vi "Mouvement encodeur.vi"(6 "Vitesse initiale":dbl, 7 "Temps acceleration":dbl, 8 "Reverse":bool, 9 "Left":bool, 10 "Right":bool, 11 "Distance":dbl) -> ()   [LabVIEW 2016]
uses:
  <vilib>/Rock Robotics/WPI/Utilities/WPI_GetSetVariantRefNum.vi
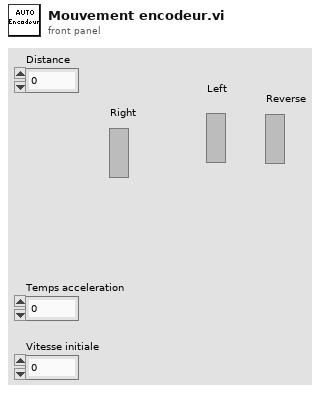
[diagram p1: front panel]
types:
  T1 = typedef "WPI_EncoderDevRef.ctl" = cluster{"DevStatus":errorcluster, "EncoderIndex":T2, "CounterIndex":T3, "DistancePerCount":dbl, "Decoding Type":T4}
  T2 = typedef "FPGA_EncoderIdx.ctl" = enum8{"Enc 0", "Enc 1", "Enc 2", "Enc 3", "Enc 4", "Enc 5", "Enc 6", "Enc 7", "Invalid"}
  T3 = typedef "FPGA_CounterCtrSystemIndex.ctl" = enum8{"Ctr 0", "Ctr 1", "Ctr 2", "Ctr 3", "Ctr 4", "Ctr 5", "Ctr 6", "Ctr 7", "Invalid"}
  T4 = typedef "WPI_EncoderType.ctl" = enum16{"1x", "2x", "4x"}
  T5 = typedef "WPI_RobotDriveDevRef.ctl" = cluster{"DevStatus":errorcluster, "Motors[]":T6[], "Square Inputs":bool, "Max Output":dbl}
  T6 = typedef "WPI_MotorControlDeviceRef.ctl" = cluster{"DeviceStatus":errorcluster, "Type":T7, "PWM":cluster{"PWM Channel":T8, "DeadBand":T9}, "CAN":cluster{"Device Number":u8, "SetOutput VI Ref":variant, "GetOutput VI Ref":variant, "Enable VI Ref":variant, "Disable VI Ref":variant, "Data":variant}, "Invert":bool}
  T7 = typedef "WPI_MotorControlType.ctl" = enum16{"PWM", "CAN"}
  T8 = typedef "FPGA_DIOPWMChannel.ctl" = enum8{"PWM 0", "PWM 1", "PWM 2", "PWM 3", "PWM 4", "PWM 5", "PWM 6", "PWM 7", "PWM 8", "PWM 9", "PWM MXP 0", "PWM MXP 1", "PWM MXP 2", "PWM MXP 3", "PWM MXP 4", "PWM MXP 5", "PWM MXP 6", "PWM MXP 7", "PWM MXP 8", "PWM MXP 9", "Invalid"}
  T9 = typedef "WPI_PWMDeadband.ctl" = cluster{"Name":string, "maxPositivePwm":i32, "minPositivePwm":i32, "centerPwm":i32, "maxNegativePwm":i32, "minNegativePwm":i32, "angularRange":u16}
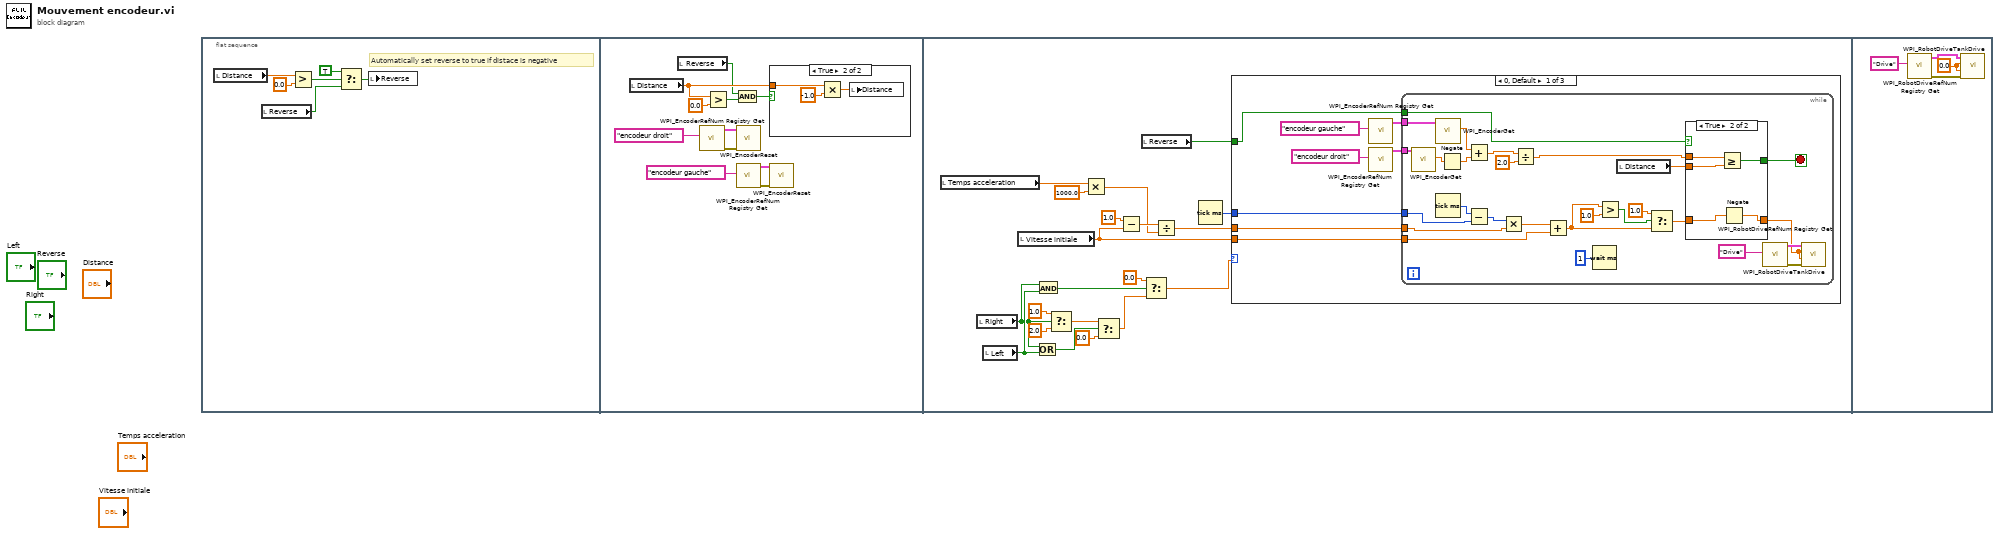
[diagram p0: block diagram]
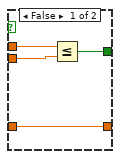
[diagram p3: hidden frame]
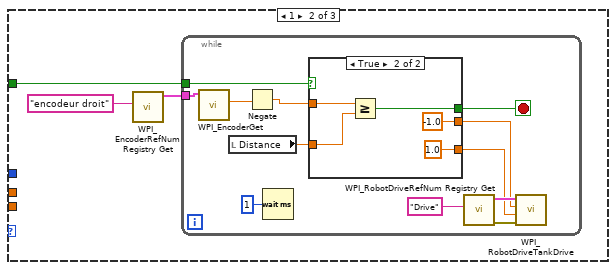
[diagram p4: hidden frame]
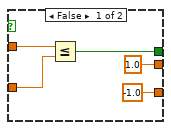
[diagram p5: hidden frame]
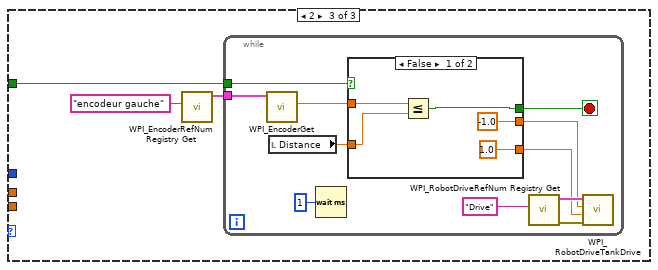
[diagram p6: hidden frame]
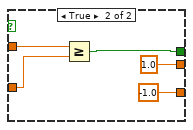
[diagram p7: hidden frame]
diagram:
  n1 = flat-sequence {
    frame #0 {
      # "Automatically set reverse to true if distace is negative"
      n2 = local read "Distance"() -> (w5:dbl)
      n3 = local read "Reverse"() -> (w3:bool)
      n4 = Greater?(x=w5, y=0.0) -> (0:w4:bool)
      n5 = Select(t=TRUE, s=w4, f=w3) -> (s? t:f=w1:bool)
      n6 = local write "Reverse"(w1) -> ()
    }
    frame #1 {
      n7 = local read "Distance"() -> (w11:dbl)
      n8 = local read "Reverse"() -> (w7:bool)
      n9 = call <vilib>:"WPI_EncoderRefNum Registry Get.vi"("refnum name"="encodeur droit") -> ("error out"=w12:errorcluster, "EncoderDevRef"=w13:T1)  [unwired: 9 in]
      n10 = Greater?(x=w11, y=0.0) -> (0:w9:bool)
      n11 = And(x=w7, y=w9) -> (x .and. y?=w10:bool)
      n12 = call <vilib>:"WPI_EncoderReset.vi"("error in (no error)"=w12, "EncoderDevRef"=w13) -> ()  [unwired: 8 in, 2 out]
      n13 = call <vilib>:"WPI_EncoderRefNum Registry Get.vi"("refnum name"="encodeur gauche") -> ("error out"=w14:errorcluster, "EncoderDevRef"=w15:T1)  [unwired: 9 in]
      n14 = case shown="True" w10 {
        tunnel: w11 -> [_ w20]
        frame False {
        }
        frame True {
          n15 = Multiply(x=w20, y=-1.0) -> (x*y=w18:dbl)
          n16 = local write "Distance"(w18) -> ()
        }
      }
      n17 = call <vilib>:"WPI_EncoderReset.vi"("error in (no error)"=w14, "EncoderDevRef"=w15) -> ()  [unwired: 8 in, 2 out]
    }
    frame #2 {
      n18 = local read "Temps acceleration"() -> (w28:dbl)
      n19 = local read "Right"() -> (w32:bool)
      n20 = local read "Left"() -> (w33:bool)
      n21 = local read "Vitesse initiale"() -> (w21:dbl)
      n22 = Or(x=w32, y=w33) -> (x .or. y?=w34:bool)
      n23 = And(x=w32, y=w33) -> (x .and. y?=w31:bool)
      n24 = Select(t=1.0, s=w32, f=2.0) -> (s? t:f=w38:dbl)
      n25 = Multiply(x=w28, y=1000.0) -> (x*y=w24:dbl)
      n26 = Select(t=w38, s=w34, f=0.0) -> (s? t:f=w35:dbl)
      n27 = Subtract(x=1.0, y=w21) -> (x-y=w25:dbl)
      n28 = local read "Reverse"() -> (w29:bool)
      n29 = Select(t=0.0, s=w31, f=w35) -> (s? t:f=w36:dbl)
      n30 = Divide(x=w25, y=w24) -> (x/y=w22:dbl)
      n31 = Tick Count (ms)() -> (millisecond timer value=w23:u32)
      n32 = case shown="0, Default" w36 {
        tunnel: w29 -> [w44 w85 w110]
        tunnel: w23 -> [w43 _ _]
        tunnel: w22 -> [w42 _ _]
        tunnel: w21 -> [w41 _ _]
        frame 0, Default {
          n33 = call <vilib>:"WPI_EncoderRefNum Registry Get.vi"("refnum name"="encodeur gauche") -> ("EncoderDevRef"=w48:T1)  [unwired: 9 in, 1 out]
          n34 = call <vilib>:"WPI_EncoderRefNum Registry Get.vi"("refnum name"="encodeur droit") -> ("EncoderDevRef"=w47:T1)  [unwired: 9 in, 1 out]
          n35 = while {
            tunnel: w47 -> [w75]
            tunnel: w48 -> [w74]
            tunnel: w44 -> [w67]
            tunnel: w43 -> [w65]
            tunnel: w42 -> [w62]
            tunnel: w41 -> [w60]
            stop <- w69 stop-if-true
            n36 = call <vilib>:"WPI_EncoderGet.vi"("EncoderDevRef"=w75) -> ("Distance"=w54:dbl)  [unwired: 5 in, 5 out]
            n37 = call <vilib>:"WPI_EncoderGet.vi"("EncoderDevRef"=w74) -> ("Distance"=w73:dbl)  [unwired: 5 in, 5 out]
            n38 = Tick Count (ms)() -> (millisecond timer value=w64:u32)
            n39 = Negate(x=w54) -> (-x=w53:dbl)
            n40 = Add(x=w73, y=w53) -> (x+y=w72:dbl)
            n41 = Subtract(x=w64, y=w65) -> (x-y=w63:u32)
            n42 = Multiply(x=w63, y=w62) -> (x*y=w61:dbl)
            n43 = Divide(x=w72, y=2.0) -> (x/y=w70:dbl)
            n44 = Add(x=w61, y=w60) -> (x+y=w57:dbl)
            n45 = Wait (ms)(milliseconds to wait=u32 1) -> ()  [unwired: 1 out]
            n46 = Greater?(x=w57, y=1.0) -> (0:w58:bool)
            n47 = local read "Distance"() -> (w68:dbl)
            n48 = Select(t=1.0, s=w58, f=w57) -> (s? t:f=w56:dbl)
            n49 = case shown="True" w67 {
              tunnel: w70 -> [w79 w84]
              tunnel: [w77 w83] -> w69
              tunnel: w68 -> [w78 w82]
              tunnel: [w76 w81] -> w49
              tunnel: w56 -> [w76 w80]
              frame False {
                n50 = Less Or Equal?(x=w79, y=w78) -> (x <= y?=w77:bool)
              }
              frame True {
                n51 = Greater Or Equal?(x=w84, y=w82) -> (x >= y?=w83:bool)
                n52 = Negate(x=w80) -> (-x=w81:dbl)
              }
            }
            n53 = call <vilib>:"WPI_RobotDriveRefNum Registry Get.vi"("refnum name"="Drive") -> ("error out"=w52:errorcluster, "RobotDriveDevRef"=w51:T5)  [unwired: 9 in]
            n54 = call <vilib>:"WPI_RobotDriveTankDrive.vi"("error in (no error)"=w52, "Right axis value"=w49, "Left axis value"=w49, "RobotDriveDevRef"=w51) -> ()  [unwired: 5 in, 3 out]
          }
        }
        frame 1 {
          n55 = call <vilib>:"WPI_EncoderRefNum Registry Get.vi"("refnum name"="encodeur droit") -> ("EncoderDevRef"=w86:T1)  [unwired: 9 in, 1 out]
          n56 = while {
            tunnel: w86 -> [w99]
            tunnel: w85 -> [w93]
            stop <- w98 stop-if-true
            n57 = call <vilib>:"WPI_EncoderGet.vi"("EncoderDevRef"=w99) -> ("Distance"=w89:dbl)  [unwired: 5 in, 5 out]
            n58 = local read "Distance"() -> (w97:dbl)
            n59 = Negate(x=w89) -> (-x=w88:dbl)
            n60 = Wait (ms)(milliseconds to wait=u32 1) -> ()  [unwired: 1 out]
            n61 = case shown="True" w93 {
              tunnel: [w102 w109] -> w98
              tunnel: w88 -> [w104 w108]
              tunnel: w97 -> [w103 w107]
              tunnel: [-1.0 ("Right axis value") 1.0 ("Right axis value")] -> w92
              tunnel: [1.0 ("Left axis value") -1.0 ("Left axis value")] -> w91
              frame False {
                n62 = Less Or Equal?(x=w104, y=w103) -> (x <= y?=w102:bool)
              }
              frame True {
                n63 = Greater Or Equal?(x=w108, y=w107) -> (x >= y?=w109:bool)
              }
            }
            n64 = call <vilib>:"WPI_RobotDriveRefNum Registry Get.vi"("refnum name"="Drive") -> ("error out"=w96:errorcluster, "RobotDriveDevRef"=w95:T5)  [unwired: 9 in]
            n65 = call <vilib>:"WPI_RobotDriveTankDrive.vi"("error in (no error)"=w96, "Right axis value"=w92, "Left axis value"=w91, "RobotDriveDevRef"=w95) -> ()  [unwired: 5 in, 3 out]
          }
        }
        frame 2 {
          n66 = call <vilib>:"WPI_EncoderRefNum Registry Get.vi"("refnum name"="encodeur gauche") -> ("EncoderDevRef"=w112:T1)  [unwired: 9 in, 1 out]
          n67 = while {
            tunnel: w112 -> [w123]
            tunnel: w110 -> [w116]
            stop <- w122 stop-if-true
            n68 = call <vilib>:"WPI_EncoderGet.vi"("EncoderDevRef"=w123) -> ("Distance"=w121:dbl)  [unwired: 5 in, 5 out]
            n69 = local read "Distance"() -> (w120:dbl)
            n70 = Wait (ms)(milliseconds to wait=u32 1) -> ()  [unwired: 1 out]
            n71 = case shown="False" w116 {
              tunnel: [w126 w133] -> w122
              tunnel: w121 -> [w128 w132]
              tunnel: w120 -> [w127 w131]
              tunnel: [-1.0 ("Left axis value") 1.0 ("Left axis value")] -> w115
              tunnel: [1.0 ("Right axis value") -1.0 ("Right axis value")] -> w114
              frame False {
                n72 = Less Or Equal?(x=w128, y=w127) -> (x <= y?=w126:bool)
              }
              frame True {
                n73 = Greater Or Equal?(x=w132, y=w131) -> (x >= y?=w133:bool)
              }
            }
            n74 = call <vilib>:"WPI_RobotDriveRefNum Registry Get.vi"("refnum name"="Drive") -> ("error out"=w117:errorcluster, "RobotDriveDevRef"=w118:T5)  [unwired: 9 in]
            n75 = call <vilib>:"WPI_RobotDriveTankDrive.vi"("error in (no error)"=w117, "Right axis value"=w114, "Left axis value"=w115, "RobotDriveDevRef"=w118) -> ()  [unwired: 5 in, 3 out]
          }
        }
      }
    }
    frame #3 {
      w137 = 0.0 ("Left axis value")
      n76 = call <vilib>:"WPI_RobotDriveRefNum Registry Get.vi"("refnum name"="Drive") -> ("error out"=w134:errorcluster, "RobotDriveDevRef"=w135:T5)  [unwired: 9 in]
      n77 = call <vilib>:"WPI_RobotDriveTankDrive.vi"("error in (no error)"=w134, "Right axis value"=w137, "Left axis value"=w137, "RobotDriveDevRef"=w135) -> ()  [unwired: 5 in, 3 out]
    }
  }
